vi "CTRE_Phoenix_MotorControl_BufferedTrajectoryPointStream_WriteAll.vi"(8 "error in":errorcluster, 10 "Motion Profile Trajectory Point Array":T1[](array[typedef]), 11 "BufferedTrajectoryPointStream_DevRef":T2) -> (0 "error out":errorcluster, 3 "BufferedTrajectoryPointStream_DevRef":T2)   [LabVIEW 2020]
doc: "Push an array of trajectory points into the Buffered Stream."
uses:
  <vilib>/Rock Robotics/WPI/ThirdParty/Phoenix-LabVIEW/Motor Controller/Controls/CTRE_Phoenix_MotorControl_BufferedTrajectoryPointStream_DeviceRef.ctl
  <vilib>/Rock Robotics/WPI/ThirdParty/Phoenix-LabVIEW/Motor Controller/Controls/CTRE_Phoenix_MotorControl_MotionProfileTrajectoryPoint.ctl
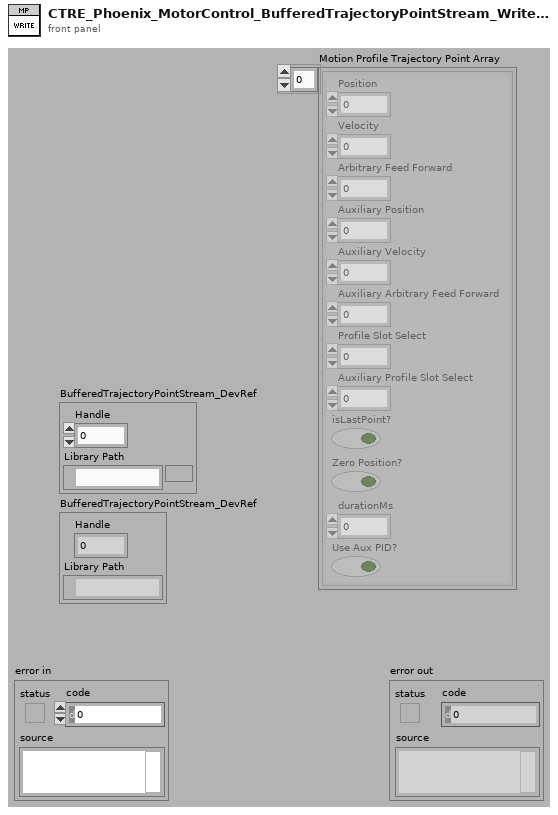
[diagram p1: front panel]
types:
  T1 = typedef "CTRE_Phoenix_MotorControl_MotionProfileTrajectoryPoint.ctl" = cluster{"Position":dbl, "Velocity":dbl, "Arbitrary Feed Forward":dbl, "Auxiliary Position":dbl, "Auxiliary Velocity":dbl, "Auxiliary Arbitrary Feed Forward":dbl, "Profile Slot Select":i32, "Auxiliary Profile Slot Select":i32, "isLastPoint?":bool, "Zero Position?":bool, "durationMs":u32, "Use Aux PID?":bool}
  T2 = typedef "CTRE_Phoenix_MotorControl_BufferedTrajectoryPointStream_DeviceRef.ctl" = cluster{"Handle":u64, "Library Path":path}
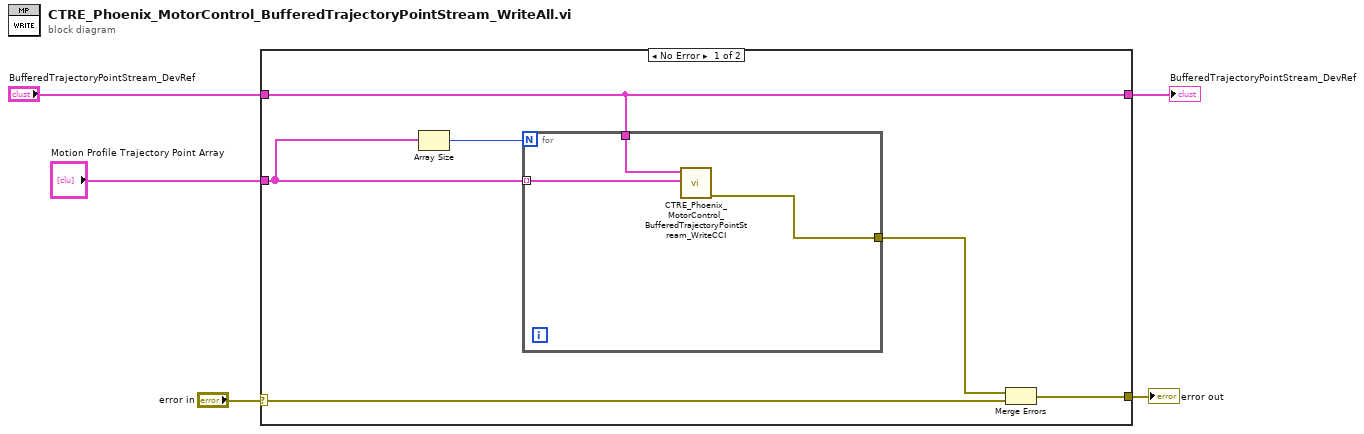
[diagram p0: block diagram]
diagram:
  n1 = case shown="No Error" "error in" {
    selector: "error in" -> [w6 w16]
    tunnel: [w7 w16] -> w5
    tunnel: [w11 w15] -> w2
    tunnel: "BufferedTrajectoryPointStream_DevRef" -> [w11 w15]
    tunnel: "Motion Profile Trajectory Point Array" -> [w9 _]
    frame No Error {
      n2 = Array Size(array=w9) -> (size(s)=w10:i32)
      n3 = for {
        N: w10 -> [_]
        tunnel: w11 -> [w14]
        tunnel: [w13] -> w8
        tunnel: w9 -> [w12] mode=indexing
        n4 = call <vilib>:"CTRE_Phoenix_MotorControl_BufferedTrajectoryPointStream_WriteCCI.vi"("Trajectory Point"=w12, "BufferedTrajectoryPointStream_DevRef"=w14) -> ("error out"=w13:errorcluster)  [unwired: 8 in, 1 out]
      }
      n5 = Merge Errors(w8, w6) -> (w7:errorcluster)
    }
    frame Error {
    }
  }
  "error out" <- w5
  "BufferedTrajectoryPointStream_DevRef" <- w2
